vi "Write SPI Digital Lines.vi"(8 "error in":errorcluster, 9 "CS Index":u8, 10 "spi output":T2, 11 "Chip Select DIO Lines":T1={"SCLK"="Port0/DIO3", "MISO"="Port0/DIO3", "MOSI"="Port0/DIO3", "CS 0"="Port0/DIO4", "CS 1"="Port0/DIO4", "CS 2"="Port0/DIO1", "CS 3"="Port0/DIO4", "CS 4"="Port0/DIO4", "CS 5"="Port0/DIO4"}) -> (0 "error out":errorcluster, 3 "Chip Select DIO Lines Out":T1={"SCLK"="Port0/DIO3", "MISO"="Port0/DIO3", "MOSI"="Port0/DIO3", "CS 0"="Port0/DIO4", "CS 1"="Port0/DIO4", "CS 2"="Port0/DIO1", "CS 3"="Port0/DIO4", "CS 4"="Port0/DIO4", "CS 5"="Port0/DIO4"})   [LabVIEW 2014]
doc: "This VI writes the user data to the MISO and SCKL and the correct CS line."
uses:
  SPI Digital IO Lines.ctl
  <userlib>/_NI SPI IP/FPGA/Controllers/Public/Spi Master Outputs.ctl
  <vilib>/rvi/eio/common/nirviEmuTemplateMethod_errors.vi
  <vilib>/eio/EIONode/EIONode.xnode
  <userlib>/_NI SPI IP/FPGA/Controllers/NI SPI IP FPGA.lvlib
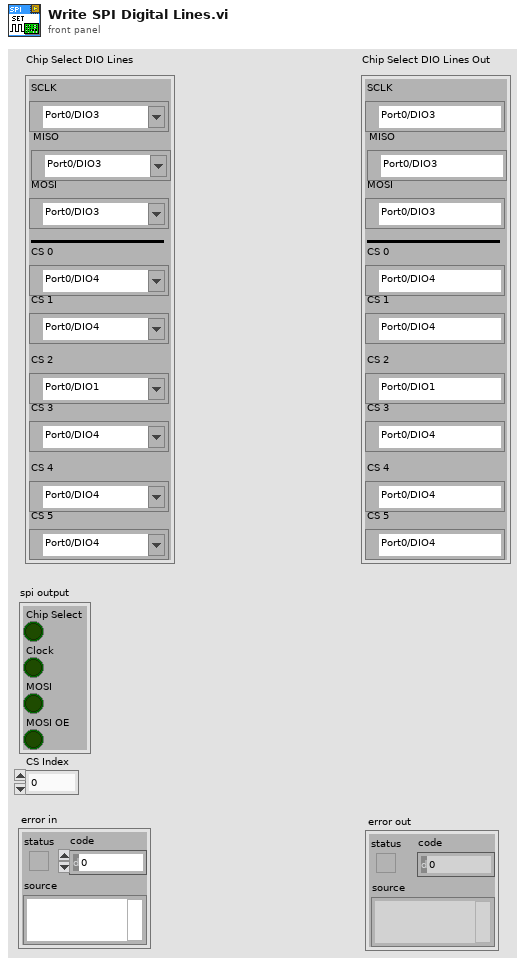
[diagram p1: front panel]
types:
  T1 = typedef "SPI Digital IO Lines.ctl" = cluster{"SCLK":refnum<k21>, "MISO":refnum<k21>, "MOSI":refnum<k21>, "CS 0":refnum<k21>, "CS 1":refnum<k21>, "CS 2":refnum<k21>, "CS 3":refnum<k21>, "CS 4":refnum<k21>, "CS 5":refnum<k21>}
  T2 = typedef "NI SPI IP FPGA.lvlib/Spi Master Outputs.ctl" = cluster{"Chip Select":bool, "Clock":bool, "MOSI":bool, "MOSI OE":bool}
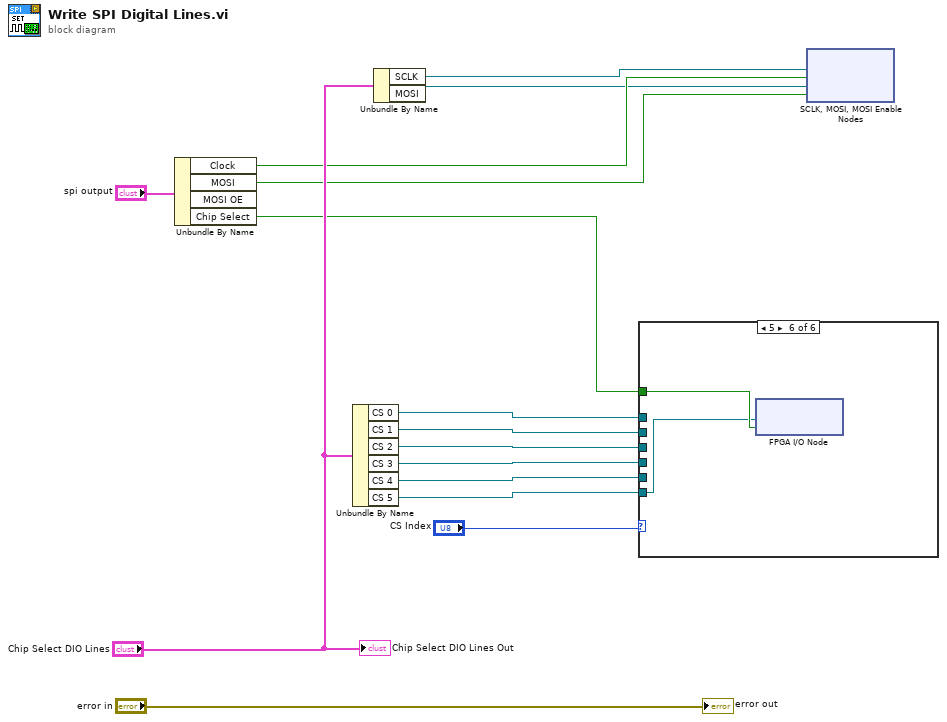
[diagram p0: block diagram]
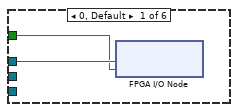
[diagram p2: hidden frame]
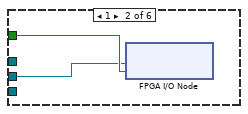
[diagram p3: hidden frame]
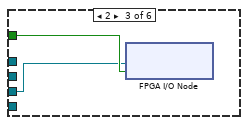
[diagram p4: hidden frame]
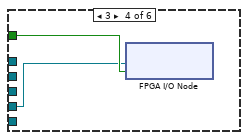
[diagram p5: hidden frame]
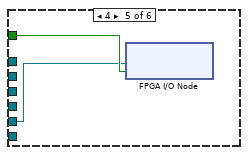
[diagram p6: hidden frame]
diagram:
  n1 = Unbundle By Name("spi output") -> ("Clock"=w11:bool, "MOSI"=w8:bool, "Chip Select"=w6:bool)  [unwired: 1 out]
  n2 = Unbundle By Name("Chip Select DIO Lines") -> ("CS 0"=w15:refnum<k21>, "CS 1"=w5:refnum<k21>, "CS 2"=w4:refnum<k21>, "CS 3"=w3:refnum<k21>, "CS 4"=w2:refnum<k21>, "CS 5"=w1:refnum<k21>)
  n3 = Unbundle By Name("Chip Select DIO Lines") -> ("SCLK"=w12:refnum<k21>, "MOSI"=w10:refnum<k21>)
  n4 = case shown="5" "CS Index" {
    tunnel: w15 -> [w17 _ _ _ _ _]
    tunnel: w6 -> [w16 w19 w21 w23 w25 w27]
    tunnel: w5 -> [_ w18 _ _ _ _]
    tunnel: w4 -> [_ _ w20 _ _ _]
    tunnel: w3 -> [_ _ _ w22 _ _]
    tunnel: w2 -> [_ _ _ _ w24 _]
    tunnel: w1 -> [_ _ _ _ _ w26]
    frame 0, Default {
      n5 = xnode "FPGA I/O Node"("I/O Item"=w16, "FPGA I/O In"=w17) -> ()  [unwired: 1 out]
    }
    frame 1 {
      n6 = xnode "FPGA I/O Node"("I/O Item"=w19, "FPGA I/O In"=w18) -> ()  [unwired: 1 out]
    }
    frame 2 {
      n7 = xnode "FPGA I/O Node"("I/O Item"=w21, "FPGA I/O In"=w20) -> ()  [unwired: 1 out]
    }
    frame 3 {
      n8 = xnode "FPGA I/O Node"("I/O Item"=w23, "FPGA I/O In"=w22) -> ()  [unwired: 1 out]
    }
    frame 4 {
      n9 = xnode "FPGA I/O Node"("I/O Item"=w25, "FPGA I/O In"=w24) -> ()  [unwired: 1 out]
    }
    frame 5 {
      n10 = xnode "FPGA I/O Node"("I/O Item"=w27, "FPGA I/O In"=w26) -> ()  [unwired: 1 out]
    }
  }
  n11 = xnode "SCLK, MOSI, MOSI Enable Nodes"("I/O Item"=w11, "FPGA I/O In"=w12, "I/O Item"=w8, "FPGA I/O In"=w10) -> ()  [unwired: 2 out]
  "error out" <- "error in"
  "Chip Select DIO Lines Out" <- "Chip Select DIO Lines"
